vi "SetPlotNameColor.vi"(8 "error in (no error)":errorcluster caption="エラー入力（エラーなし）", 9 "PlotParam":T1, 10 "PlotNo":u32, 11 "WFGraph ref in":refnum<vi>) -> (0 "error out":errorcluster caption="エラー出力", 3 "WFGraph ref out":refnum<vi>)   [LabVIEW 2015]
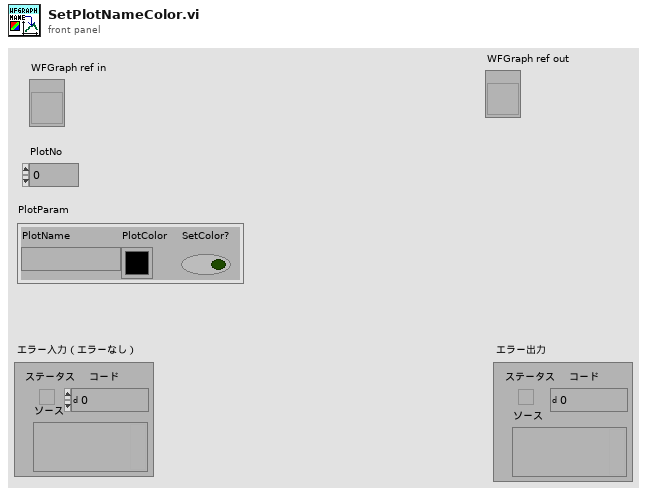
[diagram p1: front panel]
types:
  T1 = cluster{"PlotName":string, "PlotColor":u32, "SetColor?":bool}
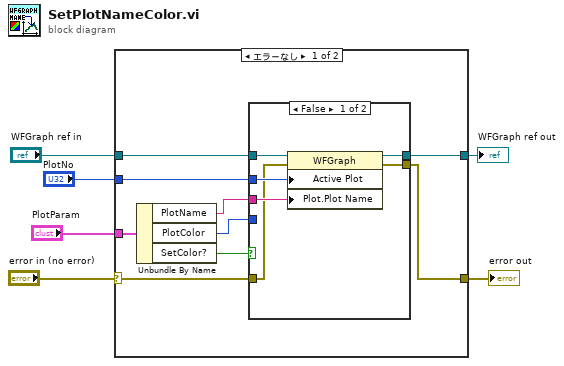
[diagram p0: block diagram]
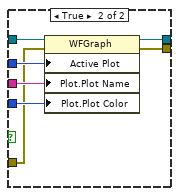
[diagram p2: hidden frame]
diagram:
  n1 = case shown="エラーなし" "error in (no error)" {
    selector: "error in (no error)" -> [w9 w30]
    tunnel: [w8 w30] -> w5
    tunnel: "WFGraph ref in" -> [w15 w29]
    tunnel: "PlotNo" -> [w14 _]
    tunnel: "PlotParam" -> [w13 _]
    tunnel: [w7 w29] -> w1
    frame No Error {
      n2 = Unbundle By Name(w13) -> ("PlotName"=w12:string, "PlotColor"=w11:u32, "SetColor?"=w10:bool)
      n3 = case shown="FALSE" w10 {
        tunnel: w15 -> [w21 w28]
        tunnel: w14 -> [w20 w27]
        tunnel: w12 -> [w19 w26]
        tunnel: w11 -> [_ w25]
        tunnel: w9 -> [w18 w24]
        tunnel: [w17 w23] -> w8
        tunnel: [w16 w22] -> w7
        frame False {
          n4 = property class="WFGraph"(reference=w21, error in=w18, "Active Plot"=w20, "Plot.Plot Name"=w19) -> (reference out=w16:refnum<vi>, error out=w17:errorcluster)
        }
        frame True {
          n5 = property class="WFGraph"(reference=w28, error in=w24, "Active Plot"=w27, "Plot.Plot Name"=w26, "Plot.Plot Color"=w25) -> (reference out=w22:refnum<vi>, error out=w23:errorcluster)
        }
      }
    }
    frame Error {
    }
  }
  "error out" <- w5
  "WFGraph ref out" <- w1
